vi "SUB_ContinueCom1Read_untilRX_empty.vi"(3 "error out 2":errorcluster, 4 "TimeOut_sec":dbl, 5 "BeginTime":u32, 6 "duplicate VISA resource name 2":refnum<visa-resource-name>) -> (0 "error out":errorcluster, 1 "String":string, 2 "duplicate VISA resource name":refnum<visa-resource-name>)   [LabVIEW 2011]
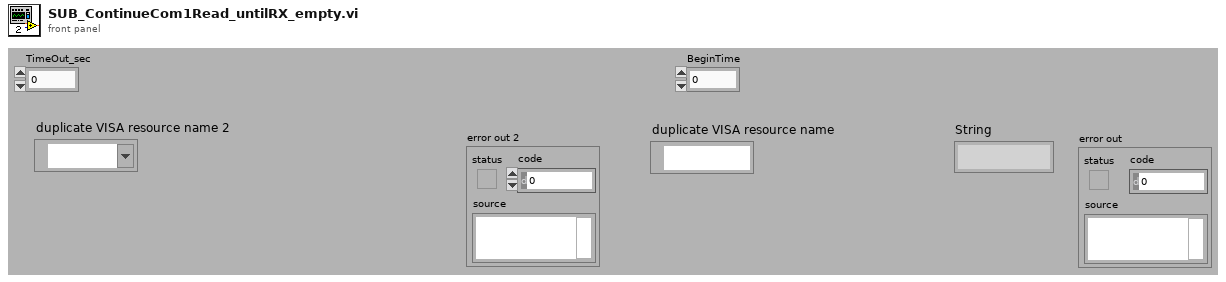
[diagram p1: front panel]
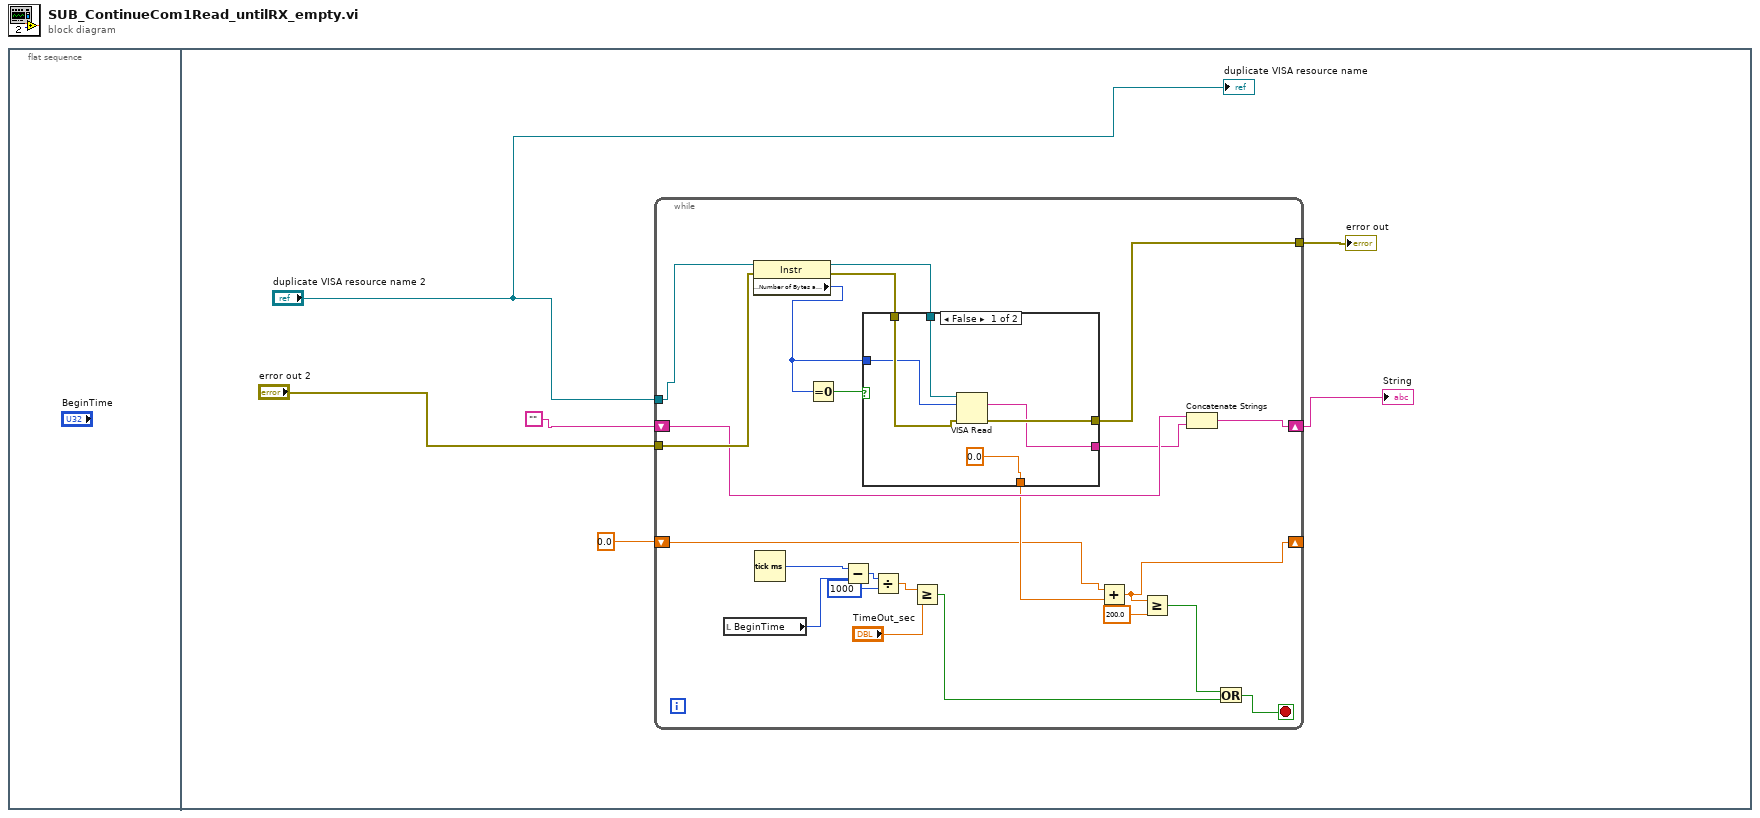
[diagram p0: block diagram]
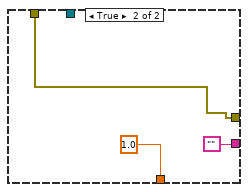
[diagram p2: hidden frame]
diagram:
  n1 = flat-sequence {
    frame #0 {
    }
    frame #1 {
      n2 = while {
        shift-right: [w21] -> w6
        shift-left: "" -> [w22]
        tunnel: "duplicate VISA resource name 2" -> [w29]
        tunnel: "error out 2" -> [w28]
        tunnel: [w23] -> w2
        shift-right: [w8] -> _
        shift-left: 0.0 ("y") -> [w7]
        stop <- w19 stop-if-true
        n3 = local read "BeginTime"() -> (w17:u32)
        n4 = property on="Property Node" class="Instr"(reference=w29, error in=w28) -> (reference out=w24:refnum<visa-resource-name>, error out=w27:errorcluster, "Serial Settings:Number of Bytes at Serial Port"=w25:u32)
        n5 = Tick Count (ms)() -> (millisecond timer value=w18:u32)
        n6 = Equal To 0?(x=w25) -> (x = 0?=w26:bool)
        n7 = Subtract(x=w18, y=w17) -> (x-y=w16:u32)
        n8 = case shown="False" w26 {
          tunnel: w27 -> [w35 w38]
          tunnel: w25 -> [w34 _]
          tunnel: w24 -> [w33 _]
          tunnel: [w32 w38] -> w23
          tunnel: [w31 ""] -> w20
          tunnel: [0.0 ("y") 1.0 ("y")] -> w9
          frame False {
            n9 = VISA Read(VISA resource name=w33, byte count=w34, error in (no error)=w35) -> (read buffer=w31:string, error out=w32:errorcluster)  [unwired: 2 out]
          }
          frame True {
          }
        }
        n10 = Divide(x=w16, y=u32 1000) -> (x/y=w14:dbl)
        n11 = Greater Or Equal?(x=w14, y="TimeOut_sec") -> (x >= y?=w13:bool)
        n12 = Add(x=w7, y=w9) -> (x+y=w8:dbl)
        n13 = Greater Or Equal?(x=w8, y=200.0) -> (x >= y?=w10:bool)
        n14 = Concatenate Strings(w22, w20) -> (w21:string)
        n15 = Or(x=w10, y=w13) -> (x .or. y?=w19:bool)
      }
      "error out" <- w2
      "String" <- w6
      "duplicate VISA resource name" <- "duplicate VISA resource name 2"
    }
  }
